vi "Test Insert Into Map.vi"() -> ()   [LabVIEW 2020]
uses:
  694f9105-211b-4265-b198-20b7d25d686f.vi
  6da77acb-fa57-4a44-a93a-8395ccd5b7d6.vi
  751aba7b-f393-4df5-a974-d29beff8fcec.vi
  <vilib>/addons/_JKI Toolkits/Caraya/classes/Assert/Assert Equal Value and Type_Variant.vi
  <vilib>/addons/_JKI Toolkits/Caraya/classes/Test/Test.lvclass
  <vilib>/addons/_JKI Toolkits/Caraya/classes/Assert/Assert.lvclass
panel:
  out "error out":errorcluster
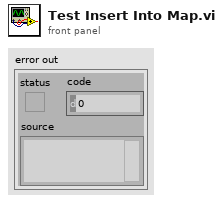
[diagram p1: front panel]
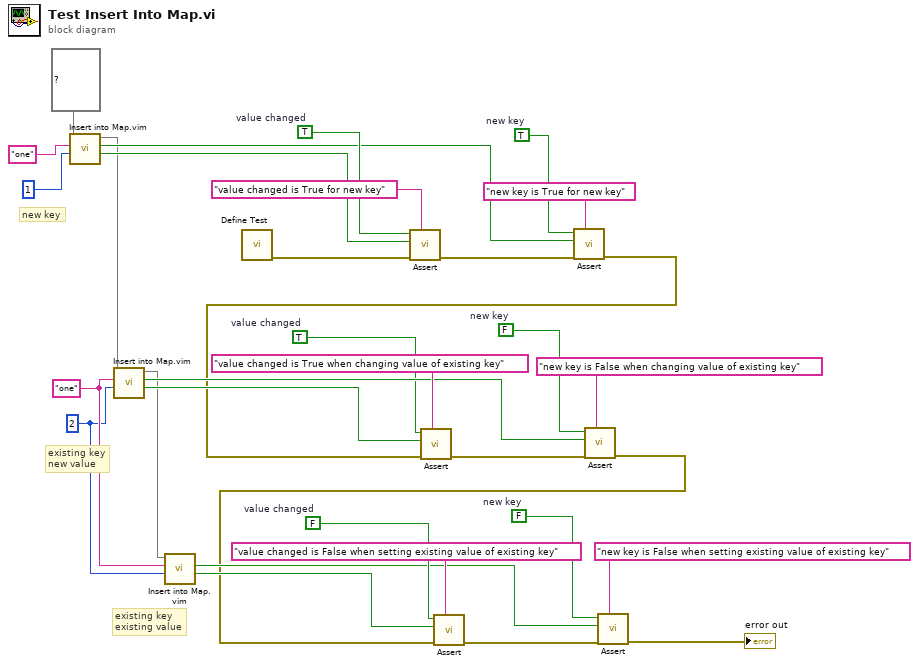
[diagram p0: block diagram]
diagram:
  w9 = FALSE  # new key
  w10 = FALSE  # value changed
  w16 = FALSE  # new key
  w15 = TRUE  # value changed
  w12 = 2 ("value type")
  w13 = "one" ("key type")
  w25 = TRUE  # new key
  w28 = TRUE  # value changed
  # "existing key\nexisting value"
  # "existing key\nnew value"
  # "new key"
  n1 = call "Insert into Map.vim"("default value"=1 ("value type"), "key"="one" ("key type"), "map"=map{string, i32} {} ("empty map")) -> ("value changed?"=w29:bool, "new key?"=w26:bool, "map out"=w22:map{string, i32})  [unwired: 6 in]
  n2 = call "Insert into Map.vim"("default value"=w12, "key"=w13, "map"=w22) -> ("value changed?"=w17:bool, "new key?"=w18:bool, "map out"=w11:map{string, i32})  [unwired: 6 in]
  n3 = call "Insert into Map.vim"("default value"=w12, "key"=w13, "map"=w11) -> ("value changed?"=w4:bool, "new key?"=w5:bool)  [unwired: 6 in, 1 out]
  n4 = call <vilib>:"Define Test.vi"() -> ("error out"=w32:errorcluster)  [unwired: 10 in, 1 out]
  n5 = call-poly <vilib>:"Assert.vi"("Label"="value changed is True for new key", "error in (no error)"=w32, "Y"=w29, "X"=w28) -> ("error out"=w27:errorcluster)  [unwired: 6 in, 1 out]
  n6 = call-poly <vilib>:"Assert.vi"("Label"="new key is True for new key", "error in (no error)"=w27, "Y"=w26, "X"=w25) -> ("error out"=w14:errorcluster)  [unwired: 6 in, 1 out]
  n7 = call-poly <vilib>:"Assert.vi"("Label"="value changed is True when changing value of existing key", "error in (no error)"=w14, "Y"=w17, "X"=w15) -> ("error out"=w19:errorcluster)  [unwired: 6 in, 1 out]
  n8 = call-poly <vilib>:"Assert.vi"("Label"="new key is False when changing value of existing key", "error in (no error)"=w19, "Y"=w18, "X"=w16) -> ("error out"=w3:errorcluster)  [unwired: 6 in, 1 out]
  n9 = call-poly <vilib>:"Assert.vi"("Label"="value changed is False when setting existing value of existing key", "error in (no error)"=w3, "Y"=w4, "X"=w10) -> ("error out"=w8:errorcluster)  [unwired: 6 in, 1 out]
  n10 = call-poly <vilib>:"Assert.vi"("Label"="new key is False when setting existing value of existing key", "error in (no error)"=w8, "Y"=w5, "X"=w9) -> ("error out"=→"error out":errorcluster)  [unwired: 6 in, 1 out]
